vi "Hardware in the Loop - Download Data (Multiplexed - Signed 16 Bit).vi"(8 "error in":errorcluster, 9 "Number of Samples":i32, 10 "Number of Channels":i32, 11 "Address":string) -> (0 "error out":errorcluster, 1 "Data Received":bool, 2 "Data":i16[][](array[numeric]))   [LabVIEW 2017, in "Communications Library.lvlib"]
doc: "Downloads multiplexed data from the DTACQ device, in 16 bit integer format, and reformats the data into a 2D array."
uses:
  Communications Library.lvlib
  Typedefs/Functional Global Variable Action--Enum.ctl
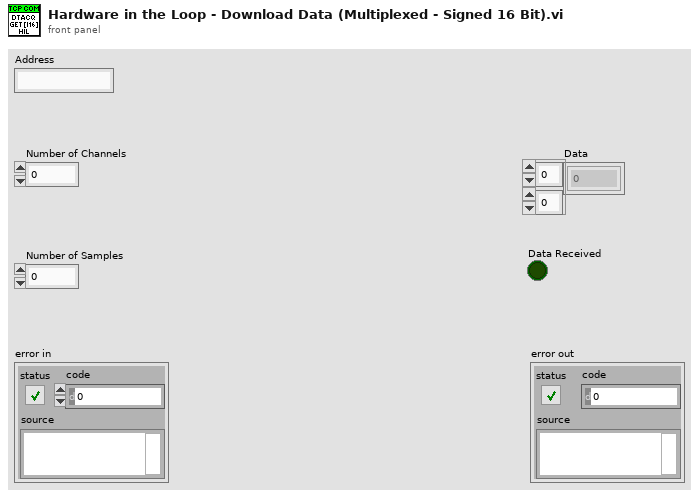
[diagram p1: front panel]
types:
  T1 = typedef "Communications Library.lvlib/Functional Global Variable Action--Enum.ctl" = enum16{"Initialise", "Write Module Config", "Write Carrier Config", "Read"}
  T2 = typedef "Communications Library.lvlib/DTACQ Module Carrier Configuration--Cluster.ctl" = cluster{"Name":string, "IP":string, "Control Port":i32, "Timeout (ms)":i32, "Continuous Capture Port (Multiplexed)":i32, "Start HIL Shot Port":i32, "AWG Upload Port (Multiplexed)":i32, "Download Captured Data Port (Multiplexed)":i32, "Module Slots":i32, "Module Configurations":T3[]}
  T3 = typedef "Communications Library.lvlib/DTACQ Module Configuration--Cluster.ctl" = cluster{"Name":string, "Position":string, "Module Type":T4, "Control Port":i32, "Timeout (ms)":i32, "Channels":i32}
  T4 = typedef "Communications Library.lvlib/DTACQ Device Type--Enum.ctl" = enum16{"Carrier", "Analog In Module", "Analog Out Module", "Generic Module"}
  T5 = typedef "Communications Library.lvlib/DTACQ Connection Data--Cluster.ctl" = cluster{"Description":string, "Address":string, "Port":u16, "timeout (ms)":i32, "Termination Character":string, "TCP Connection Reference":refnum<k5>, "Open Connection":bool}
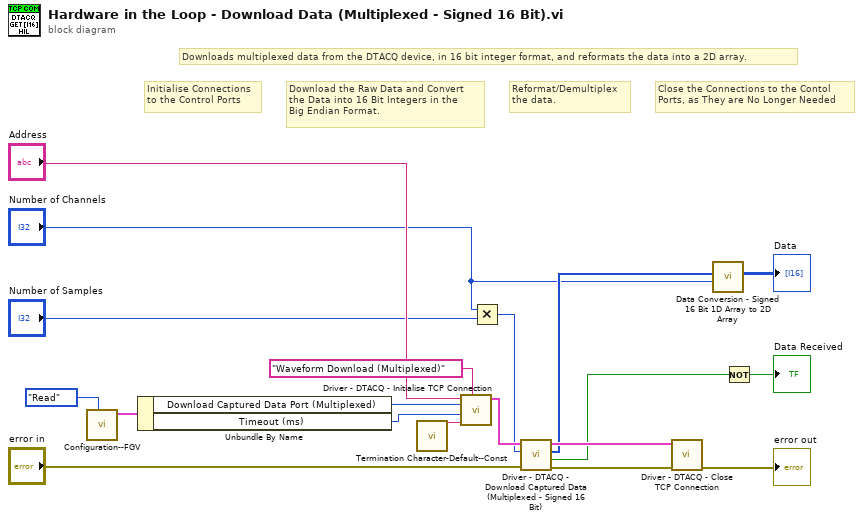
[diagram p0: block diagram]
diagram:
  # "Downloads multiplexed data from the DTACQ device, in 16 bit integer format, and reformats the data into a 2D array."
  # "Close the Connections to the Contol\nPorts, as They are No Longer Needed"
  # "Reformat/Demultiplex\nthe data."
  # "Download the Raw Data and Convert\nthe Data into 16 Bit Integers in the\nBig Endian Format."
  # "Initialise Connections\nto the Control Ports"
  n1 = call "Configuration--FGV.vi"("Functional Global Action"=Functional_Global_Variable_Action--Enum."Read") -> ("Carrier Configuration Out"=w3:T2)  [unwired: 9 in, 1 out]
  n2 = Unbundle By Name(w3) -> ("Download Captured Data Port (Multiplexed)"=w2:i32, "Timeout (ms)"=w1:i32)
  n3 = call "Termination Character-Default--Const.vi"() -> ("Termination Character"=w9:string)  [unwired: 11 in]
  n4 = call "Driver - DTACQ - Initialise TCP Connection.vi"("Description"="Waveform Download (Multiplexed)", "Termination Character"=w9, "timeout (ms)"=w1, "Port"=w2, "Address"="Address") -> ("DTACQ Connection Data Out"=w18:T5)  [unwired: 6 in]
  n5 = Multiply(x="Number of Channels", y="Number of Samples") -> (x*y=w8:i32)
  n6 = call "Driver - DTACQ - Download Captured Data (Multiplexed - Signed 16 Bit).vi"("error in"="error in", "Samples"=w8, "DTACQ Connection Data In"=w18) -> ("error out"=w13:errorcluster, "Timed Out"=w12:bool, "(Signed) 16 Bit Array"=w6:i16[], "DTACQ Connection Data Out"=w17:T5)  [unwired: 5 in]
  n7 = call "Driver - DTACQ - Close TCP Connection.vi"("error in"=w13, "DTACQ Connection Data In"=w17) -> ("error out"=→"error out":errorcluster)  [unwired: 8 in, 1 out]
  n8 = call "Data Conversion - Signed 16 Bit 1D Array to 2D Array.vi"("Channels"="Number of Channels", "1D Data (Multiplexed)"=w6) -> ("2D Data (De-Multiplexed)"=→"Data":i16[][])  [unwired: 9 in]
  n9 = Not(x=w12) -> (.not. x?=→"Data Received":bool)
